vi "CPU_calc_speed.vi"(10 "clock ticks":u32) -> (2 "clock ticks out":u32, 3 "ticks/s":u32 format="%.2p")   [LabVIEW 2018]
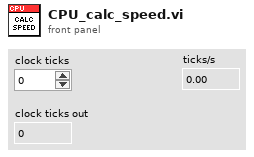
[diagram p1: front panel]
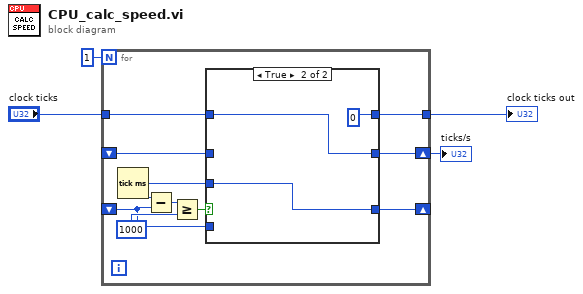
[diagram p0: block diagram]
diagram:
  n1 = for {
    N: 1 -> [_]
    tunnel: "clock ticks" -> [w9]
    shift-right: [w10] -> _
    shift-left: _ -> [w8]
    shift-right: [w7] -> w2
    shift-left: _ -> [w6]
    tunnel: [w5] -> w1
    n2 = Tick Count (ms)() -> (millisecond timer value=w11:u32)
    n3 = Subtract(x=w11, y=w8) -> (x-y=w14:u32)
    n4 = Greater Or Equal?(x=w14, y=u32 1000) -> (x >= y?=w12:bool)
    n5 = case shown="True" w12 {
      tunnel: w11 -> [_ w20]
      tunnel: [w17 w20] -> w10
      tunnel: w9 -> [w15 w18]
      tunnel: w8 -> [w17 _]
      tunnel: [w16 w18] -> w7
      tunnel: w6 -> [w16 _]
      tunnel: [w15 u32 0] -> w5
      frame False {
      }
      frame True {
      }
    }
  }
  "ticks/s" <- w2
  "clock ticks out" <- w1
